vi "MGCC_MdlMgmt_Feeder.vi"() -> ()   [LabVIEW 2016]
doc: "-----------------------------------------------------------------------------------------------------------------------\nCopyright <2019> <The University of Tennessee at Knoxville and the University of Tennessee Research Foundation>\nThis software is released under BSD-3 \nhttps://opensource.org/licenses/BSD-3-Clause \nAdditional license options available at https://utrf.tennessee.edu/industry/sample-agreements/\n-----------------------------------------------------------------------------------------------------------------------"
uses:
  <vilib>/imath/engines/lvmath2/RunTimeEngine/RunTimeType/NIMS_RunTimeType_From StrictType (excl LVString).vi
  <instcachedir>/0/NIMS_RunTimeType_From StrictType (excl LVString)_BBF44FB49F834B71AF7A14CCEDF8BECD.lvgen/NIMS_RunTimeType_From StrictType (excl LVString)_BBF44FB49F834B71AF7A14CCEDF8BECD_009.vi
  <vilib>/imath/engines/lvmath2/RunTimeEngine/Struct/NIMS_StructSetField.vi
  <instcachedir>/0/NIMS_RunTimeType_From StrictType (excl LVString)_BBF44FB49F834B71AF7A14CCEDF8BECD.lvgen/NIMS_RunTimeType_From StrictType (excl LVString)_BBF44FB49F834B71AF7A14CCEDF8BECD_031.vi
  <instcachedir>/0/NIMS_RunTimeType_From StrictType (excl LVString)_BBF44FB49F834B71AF7A14CCEDF8BECD.lvgen/NIMS_RunTimeType_From StrictType (excl LVString)_BBF44FB49F834B71AF7A14CCEDF8BECD_007.vi
  <instcachedir>/0/NIMS_RunTimeType_From StrictType (excl LVString)_BBF44FB49F834B71AF7A14CCEDF8BECD.lvgen/NIMS_RunTimeType_From StrictType (excl LVString)_BBF44FB49F834B71AF7A14CCEDF8BECD_010.vi
  <vilib>/imath/engines/lvmath2/RunTimeEngine/Struct/NIMS_StructGetField.vi
  <vilib>/imath/engines/lvmath2/RunTimeEngine/RunTimeType/NIMS_RunTimeType_To Numeric.vi
  <instcachedir>/0/NIMS_RunTimeType_To Numeric_19D51BCABB82435A94073491761E42EE.lvgen/NIMS_RunTimeType_To Numeric_19D51BCABB82435A94073491761E42EE_004.vi
  <instcachedir>/0/NIMS_RunTimeType_To Numeric_19D51BCABB82435A94073491761E42EE.lvgen/NIMS_RunTimeType_To Numeric_19D51BCABB82435A94073491761E42EE_009.vi
  <instcachedir>/0/NIMS_RunTimeType_To Numeric_19D51BCABB82435A94073491761E42EE.lvgen/NIMS_RunTimeType_To Numeric_19D51BCABB82435A94073491761E42EE_003.vi
  <instcachedir>/0/NIMS_RunTimeType_To Numeric_19D51BCABB82435A94073491761E42EE.lvgen/NIMS_RunTimeType_To Numeric_19D51BCABB82435A94073491761E42EE_002.vi
  <vilib>/imath/engines/lvmath2/RunTimeEngine/NodeEndStatement/NIMS_NodeEndStatement_Output.vi
  <instcachedir>/0/NIMS_NodeEndStatement_Output_53EC0D466D134D7ABD903AC30B43404B.lvgen/NIMS_NodeEndStatement_Output_53EC0D466D134D7ABD903AC30B43404B_028.vi
  <vilib>/imath/engines/lvmath2/RunTimeEngine/ErrorHandling/NIMS_Finalize Error.vi
panel:
  out "output cluster":T1
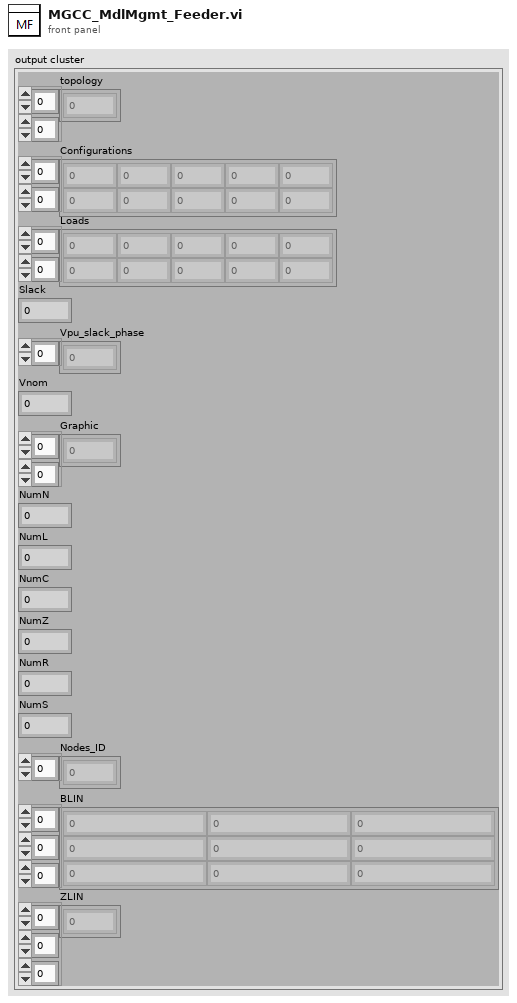
[diagram p1: front panel]
types:
  T1 = cluster{"topology":dbl[][], "Configurations":dbl[][], "Loads":dbl[][], "Slack":dbl, "Vpu_slack_phase":cdb[], "Vnom":dbl, "Graphic":dbl[][], "NumN":dbl, "NumL":dbl, "NumC":dbl, "NumZ":dbl, "NumR":dbl, "NumS":dbl, "Nodes_ID":dbl[], "BLIN":cdb[][][], "ZLIN":cdb[][][]}
  T2 = cluster{"Topology":dbl[][], "Configurations":dbl[][], "Loads":dbl[][], "Slack":dbl, "Vpu_slack_phase":cdb[], "Vnom":dbl, "Graphic":dbl[][], "NumN":dbl, "NumL":dbl, "NumC":dbl, "NumZ":dbl, "NumR":dbl, "NumS":dbl, "Nodes_ID":dbl[]}
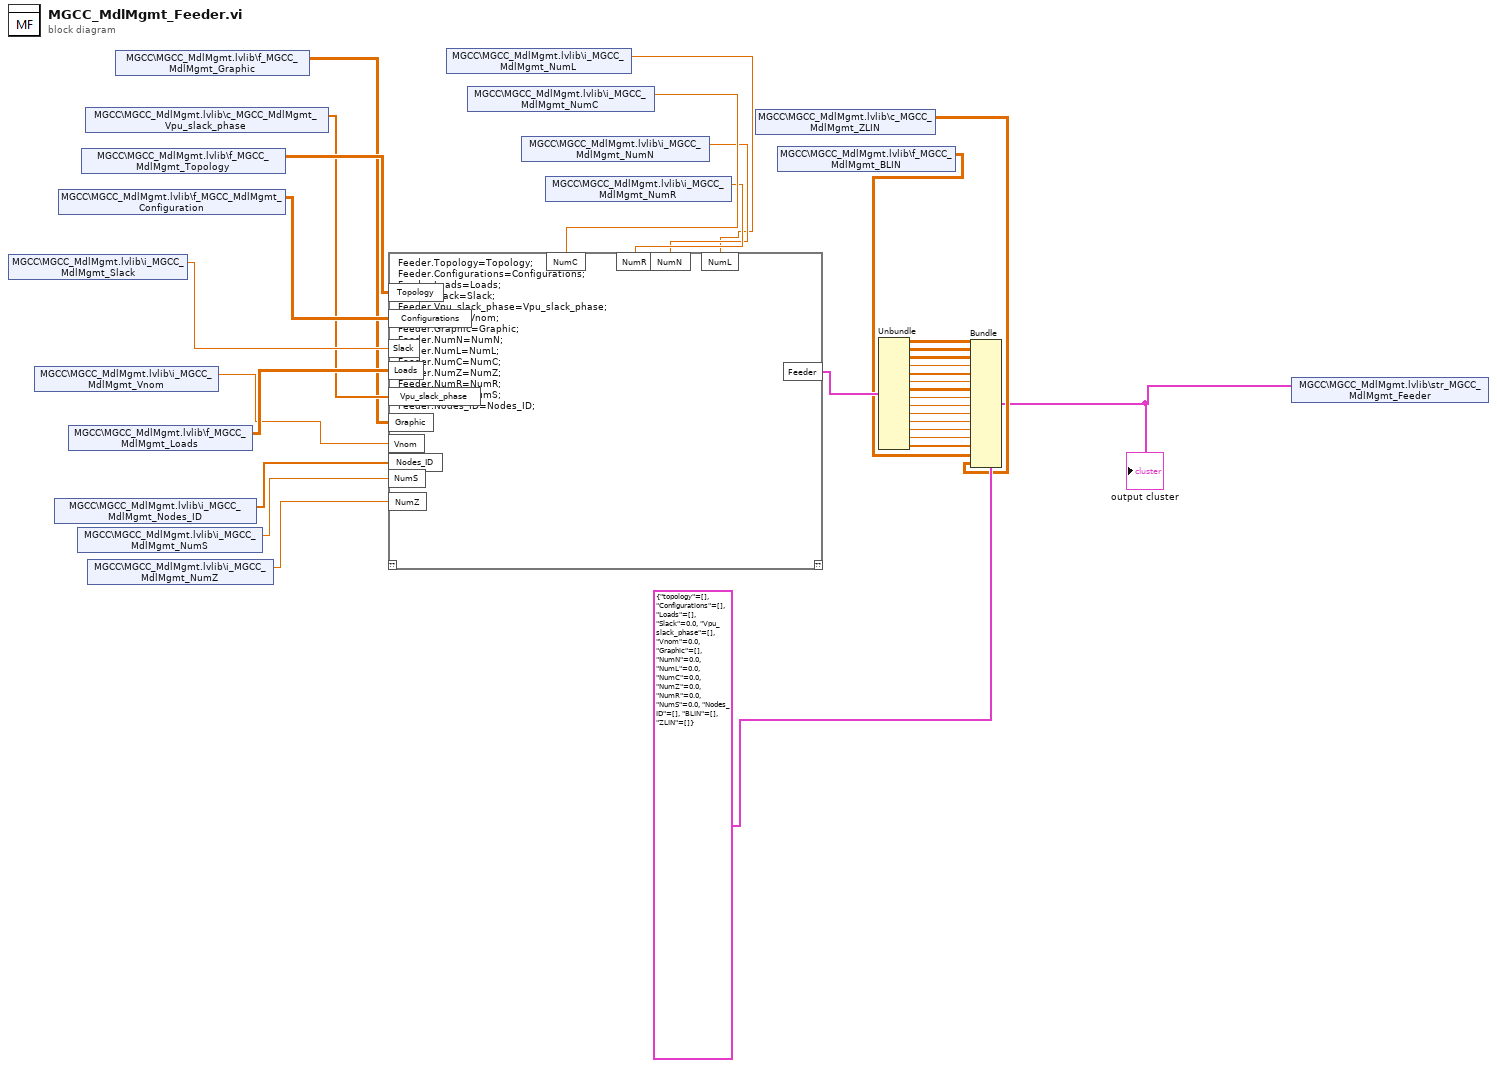
[diagram p0: block diagram]
diagram:
  n1 = shared-variable "MGCC\\MGCC_MdlMgmt.lvlib\\i_MGCC_MdlMgmt_Slack"() -> (w31:dbl)  [unwired: 1 in, 1 out]
  n2 = shared-variable "MGCC\\MGCC_MdlMgmt.lvlib\\i_MGCC_MdlMgmt_Vnom"() -> (w27:dbl)  [unwired: 1 in, 1 out]
  n3 = shared-variable "MGCC\\MGCC_MdlMgmt.lvlib\\i_MGCC_MdlMgmt_Nodes_ID"() -> (w26:dbl[])  [unwired: 1 in, 1 out]
  n4 = shared-variable "MGCC\\MGCC_MdlMgmt.lvlib\\f_MGCC_MdlMgmt_Configuration"() -> (w32:dbl[][])  [unwired: 1 in, 1 out]
  n5 = shared-variable "MGCC\\MGCC_MdlMgmt.lvlib\\f_MGCC_MdlMgmt_Loads"() -> (w30:dbl[][])  [unwired: 1 in, 1 out]
  n6 = shared-variable "MGCC\\MGCC_MdlMgmt.lvlib\\i_MGCC_MdlMgmt_NumS"() -> (w25:dbl)  [unwired: 1 in, 1 out]
  n7 = shared-variable "MGCC\\MGCC_MdlMgmt.lvlib\\f_MGCC_MdlMgmt_Topology"() -> (w33:dbl[][])  [unwired: 1 in, 1 out]
  n8 = shared-variable "MGCC\\MGCC_MdlMgmt.lvlib\\c_MGCC_MdlMgmt_Vpu_slack_phase"() -> (w29:cdb[])  [unwired: 1 in, 1 out]
  n9 = shared-variable "MGCC\\MGCC_MdlMgmt.lvlib\\i_MGCC_MdlMgmt_NumZ"() -> (w24:dbl)  [unwired: 1 in, 1 out]
  n10 = shared-variable "MGCC\\MGCC_MdlMgmt.lvlib\\f_MGCC_MdlMgmt_Graphic"() -> (w28:dbl[][])  [unwired: 1 in, 1 out]
  n11 = shared-variable "MGCC\\MGCC_MdlMgmt.lvlib\\i_MGCC_MdlMgmt_NumL"() -> (w20:dbl)  [unwired: 1 in, 1 out]
  n12 = shared-variable "MGCC\\MGCC_MdlMgmt.lvlib\\i_MGCC_MdlMgmt_NumC"() -> (w23:dbl)  [unwired: 1 in, 1 out]
  n13 = shared-variable "MGCC\\MGCC_MdlMgmt.lvlib\\i_MGCC_MdlMgmt_NumN"() -> (w21:dbl)  [unwired: 1 in, 1 out]
  n14 = shared-variable "MGCC\\MGCC_MdlMgmt.lvlib\\i_MGCC_MdlMgmt_NumR"() -> (w22:dbl)  [unwired: 1 in, 1 out]
  n15 = mathscript code="Feeder.Topology=Topology;\nFeeder.Configurations=Configurations;\nFeeder.Loads=Loads;\nFeeder.Slack=Slack;\nFeeder.Vpu_slack_phase=Vpu_slack_phase;\nFeeder.Vnom=Vnom;\nFeeder.Graphic=Graphic;\nFeeder.NumN=NumN;\nFeeder.NumL=NumL;\nFeeder.NumC=NumC;\nFeeder.NumZ=NumZ;\nFeeder.NumR=NumR;\nFeeder.NumS=NumS;\nFeeder.Nodes_ID=Nodes_ID;"("Topology"=w33, "Configurations"=w32, "Slack"=w31, "Loads"=w30, "Vpu_slack_phase"=w29, "Graphic"=w28, "Vnom"=w27, "Nodes_ID"=w26, "NumS"=w25, "NumZ"=w24, "NumC"=w23, "NumR"=w22, "NumN"=w21, "NumL"=w20) -> ("Feeder"=w18:T2)  [unwired: 1 in, 1 out]
  n16 = shared-variable "MGCC\\MGCC_MdlMgmt.lvlib\\c_MGCC_MdlMgmt_ZLIN"() -> (w2:cdb[][][])  [unwired: 1 in, 1 out]
  n17 = shared-variable "MGCC\\MGCC_MdlMgmt.lvlib\\f_MGCC_MdlMgmt_BLIN"() -> (w3:cdb[][][])  [unwired: 1 in, 1 out]
  n18 = Unbundle(w18) -> ("Topology"=w17:dbl[][], "Configurations"=w16:dbl[][], "Loads"=w15:dbl[][], "Slack"=w14:dbl, "Vpu_slack_phase"=w13:cdb[], "Vnom"=w12:dbl, "Graphic"=w11:dbl[][], "NumN"=w10:dbl, "NumL"=w9:dbl, "NumC"=w8:dbl, "NumZ"=w7:dbl, "NumR"=w6:dbl, "NumS"=w5:dbl, "Nodes_ID"=w4:dbl[])
  n19 = Bundle(cluster=T1 {"topology"=[], "Configurations"=[], "Loads"=[], "Slack"=0.0, "Vpu_slack_phase"=[], "Vnom"=0.0, "Graphic"=[], "NumN"=0.0, "NumL"=0.0, "NumC"=0.0, "NumZ"=0.0, "NumR"=0.0, "NumS"=0.0, "Nodes_ID"=[], "BLIN"=[], "ZLIN"=[]} ("str_MGCC_MdlMgmt_Feeder"), "topology"=w17, "Configurations"=w16, "Loads"=w15, "Slack"=w14, "Vpu_slack_phase"=w13, "Vnom"=w12, "Graphic"=w11, "NumN"=w10, "NumL"=w9, "NumC"=w8, "NumZ"=w7, "NumR"=w6, "NumS"=w5, "Nodes_ID"=w4, "BLIN"=w3, "ZLIN"=w2) -> (w1:T1)
  "output cluster" <- w1
  n20 = shared-variable "MGCC\\MGCC_MdlMgmt.lvlib\\str_MGCC_MdlMgmt_Feeder"(w1) -> ()  [unwired: 1 in, 1 out]
